vi "EZDA.vi"() -> ()   [LabVIEW 2018]
panel:
  in  "Серво":dbl(knob) scale=0.0..0.13
  in  "Подъемник":dbl(slide) scale=100.0..-100.0
  in  "Остановка":bool
  in  "Направо":bool
  in  "Налево":bool
  in  "Вперед":bool
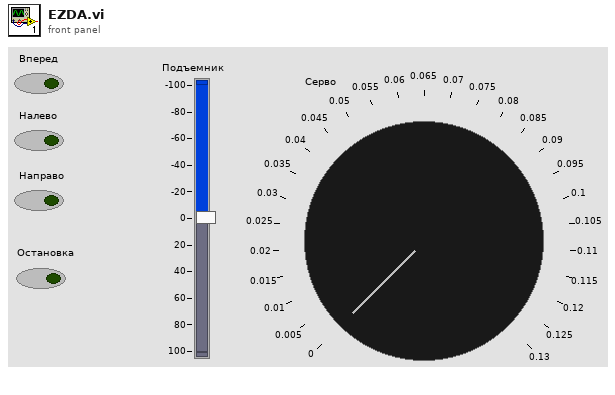
[diagram p1: front panel]
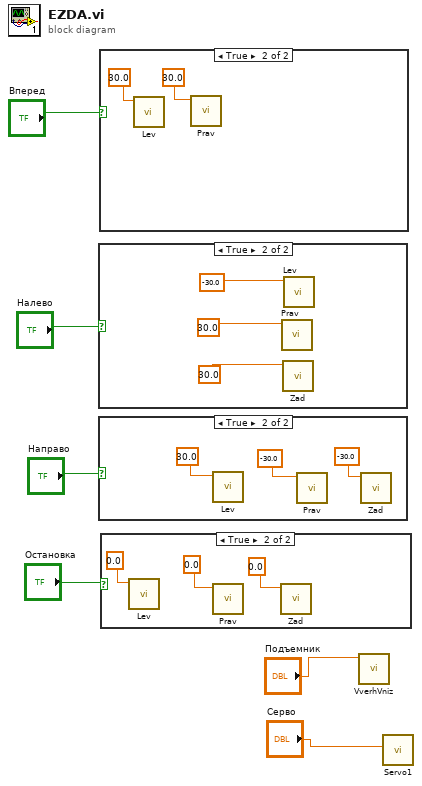
[diagram p0: block diagram]
diagram:
  n1 = case shown="True" "Налево" {
    frame False {
    }
    frame True {
      n2 = call "Prav.vi"("Numeric"=30.0) -> ()  [unwired: 10 in, 1 out]
      n3 = call "Zad.vi"("Numeric"=30.0) -> ()  [unwired: 10 in, 1 out]
      n4 = call "Lev.vi"("Numeric"=-30.0) -> ()  [unwired: 10 in, 1 out]
    }
  }
  n5 = case shown="True" "Направо" {
    frame False {
    }
    frame True {
      n6 = call "Lev.vi"("Numeric"=30.0) -> ()  [unwired: 10 in, 1 out]
      n7 = call "Prav.vi"("Numeric"=-30.0) -> ()  [unwired: 10 in, 1 out]
      n8 = call "Zad.vi"("Numeric"=-30.0) -> ()  [unwired: 10 in, 1 out]
    }
  }
  n9 = case shown="True" "Вперед" {
    frame False {
    }
    frame True {
      n10 = call "Lev.vi"("Numeric"=30.0) -> ()  [unwired: 10 in, 1 out]
      n11 = call "Prav.vi"("Numeric"=30.0) -> ()  [unwired: 10 in, 1 out]
    }
  }
  n12 = case shown="True" "Остановка" {
    frame False {
    }
    frame True {
      n13 = call "Lev.vi"("Numeric"=0.0) -> ()  [unwired: 10 in, 1 out]
      n14 = call "Prav.vi"("Numeric"=0.0) -> ()  [unwired: 10 in, 1 out]
      n15 = call "Zad.vi"("Numeric"=0.0) -> ()  [unwired: 10 in, 1 out]
    }
  }
  n16 = call "VverhVniz.vi"("Numeric"="Подъемник") -> ()  [unwired: 10 in, 1 out]
  n17 = call "Servo1.vi"("Knob"="Серво") -> ()  [unwired: 10 in, 1 out]
